vi "Read Response ADC.vi"(8 "error in (no error)":errorcluster, 11 "Simulado in":refnum<class "Simulado.lvclass">) -> (0 "error out":errorcluster, 2 "Respuesta":string, 3 "Simulado out":refnum<class "Simulado.lvclass">)   [LabVIEW 2020, in "Simulado.lvclass"]
uses:
  Simulado.lvclass
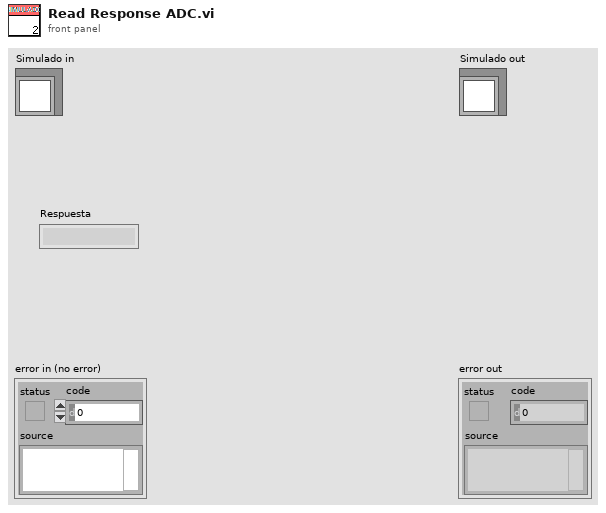
[diagram p1: front panel]
types:
  T1 = enum16{"reset parameters", "Get parameters", "Set parameter"}
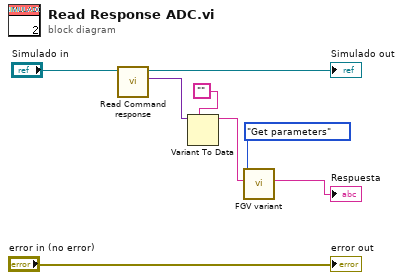
[diagram p0: block diagram]
diagram:
  n1 = call-dynamic "Read Command response.vi"("Simulado in"="Simulado in") -> ("Command response"=w4:variant, "Simulado out"=→"Simulado out":refnum<class "Simulado.lvclass">)  [unwired: 8 in, 1 out]
  n2 = Variant To Data(type="", Variant=w4) -> (data=w2:string)  [unwired: 1 in, 1 out]
  n3 = call "FGV variant.vi"("Command"=w2, "Functions"=T1."Get parameters") -> ("Response retrieved"=→"Respuesta":string)  [unwired: 8 in, 1 out]
  "error out" <- "error in (no error)"
